vi "Get From Symbol Map.vi"(8 "error in (no error)":errorcluster, 10 "Symbol Name":string, 11 "TwinCAT ADS in":refnum<class "TwinCAT ADS.lvclass">) -> (0 "error out":errorcluster, 1 ".NET Symbol Information":refnum<k24>, 2 "Found?":bool, 3 "TwinCAT ADS out":refnum<class "TwinCAT ADS.lvclass">)   [LabVIEW 2018, in "TwinCAT ADS.lvclass"]
uses:
  TwinCAT ADS.lvclass
  TwinCAT.Ads
  TwinCAT ADS.lvclass/TwinCAT ADS.ctl
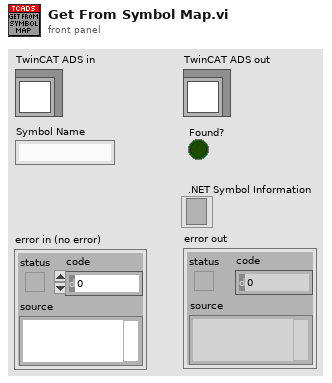
[diagram p1: front panel]
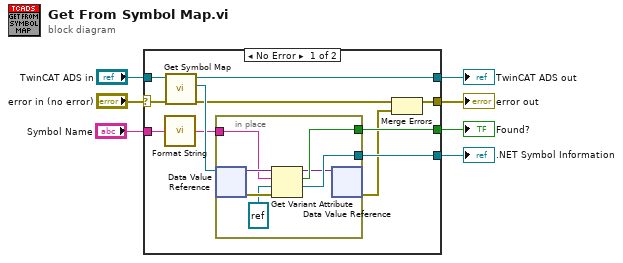
[diagram p0: block diagram]
diagram:
  n1 = case shown="No Error" "error in (no error)" {
    selector: "error in (no error)" -> [w12 w26]
    tunnel: "TwinCAT ADS in" -> [w18 w27]
    tunnel: "Symbol Name" -> [w16 _]
    tunnel: [w10 w26] -> w5
    tunnel: [w14 w27] -> w4
    tunnel: [w13 _] -> w2
    tunnel: [w9 _] -> w1
    frame No Error {
      n2 = call "Format String.vi"("String"=w16) -> ("Formated String"=w15:string)
      n3 = call "Get Symbol Map.vi"("error in (no error)"=w12, "TwinCAT ADS in"=w18) -> ("error out"=w11:errorcluster, "Symbol Map"=w17:refnum<data-value>, "TwinCAT ADS out"=w14:refnum<class "TwinCAT ADS.lvclass">)  [unwired: 7 in]
      n4 = in-place {
        in-place-border: w15 -> [w23]
        in-place-border: [w21] -> w9
        in-place-border: [w20] -> w13
        n5 = in-place-dvr #1(w17) -> (w24:variant, w25:errorcluster)
        n6 = Get Variant Attribute(Variant=w24, name=w23, default value (empty Variant)=refnum<k24> refnum (".NET Symbol Information"), error in=w25) -> (duplicate Variant=w19:variant, found=w20:bool, value=w21:refnum<k24>)  [unwired: 1 out]
        n7 = in-place-dvr #1(w19) -> (w8:errorcluster)  [unwired: 1 out]
      }
      n8 = Merge Errors(w11, w8) -> (w10:errorcluster)
    }
    frame Error {
    }
  }
  "error out" <- w5
  "TwinCAT ADS out" <- w4
  ".NET Symbol Information" <- w1
  "Found?" <- w2
